vi "Digital Patterns Page.vi"(8 "error in (no error)":errorcluster, 11 "Node Ptr":T1 format="%.0x") -> (0 "error out":errorcluster)   [LabVIEW 2015, in "Engine Simulation Toolkit System Explorer.lvlib"]
uses:
  Engine Simulation Toolkit System Explorer.lvlib
  <vilib>/NI Veristand/Custom Device API/Custom Device Item Ref.ctl
  Digital Patterns Page Data.ctl
  Digital Pattern.ctl
  Digital Pattern Base.ctl
  Digital Pattern Remove Edge.ctl
  Digital Pattern Add Pulse.ctl
  File Formats.lvlibp/Parent/EST Pattern.ctl
  Shared/Properties.vi
  Shared/Constants and GUIDs.vi
  <vilib>/NI Veristand/Custom Device API/Custom Device API.lvlib
  Shared/Engine Simulation Toolkit Shared.lvlib
  <vilib>/NI/GXML/GXML.lvlib
  File Formats.lvlibp/Parent/FileFormat.lvclass
panel:
  in  "FPGA Resource":u16(ring) items=["Select an item..."]
  in  "pattern_remove":bool
  in  "pattern_add":bool caption="remove_add"
  in  "add_add":bool caption="remove_add"
  in  "Chart_Offset":dbl caption="Offset" format="%#_6f"
  in  "Chart_Tooth":u16 caption="Tooth"
  in  "Chart_Position":dbl caption="Position" format="%#_6f"
  in  "Edge":bool
  in  "remove_Tooth":u16 caption="Start\nTooth"
  in  "add_Offset":dbl caption="Offset"
  in  "add_Width":dbl caption="Width"
  in  "add_Tooth":u16 caption="Tooth"
  in  "base_Offset":dbl caption="Offset"
  in  "base_Toothwidth":dbl caption="Tooth width"
  in  "base_teeth":u16 caption="Teeth"
  in  "base_Length":dbl caption="Length"
  in  "add_remove":bool
  in  "remove_remove":bool
  in  "remove_add":bool
  in  "Pattern Name":string caption="Name"
  in  "Edges Removed":i32(listbox)
  in  "Pulses Added":i32(listbox)
  in  "Patterns":i32[](listbox)
  in  "Zoom":cluster{dbl, dbl}(slide)={360.0, -360.0} scale=-360.0..360.0
  out "Pattern Plot":cluster{dbl[], dbl[]}[](graph)
  in  "Header":cluster{"Section Name":string}={"Section Name"="Digital Patterns Settings"}
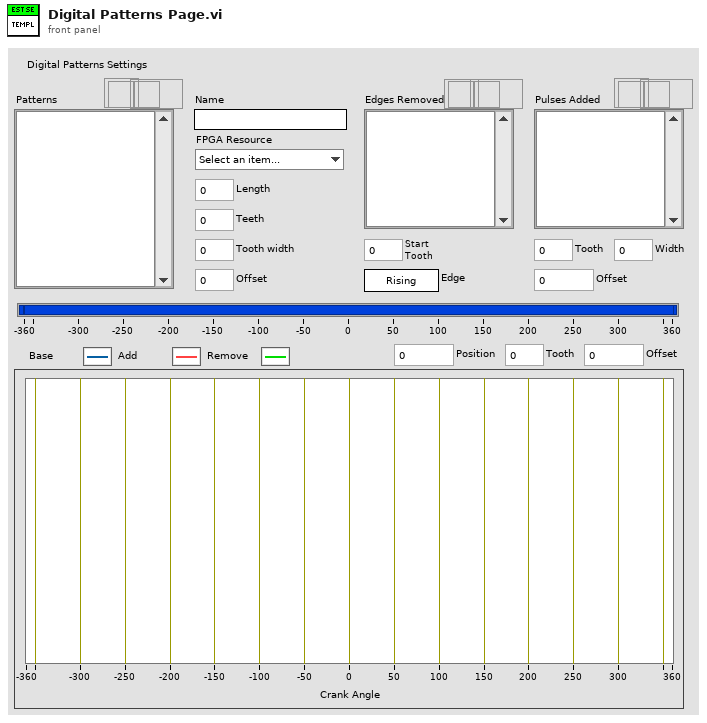
[diagram p1: front panel]
types:
  T1 = typedef "Custom Device API.lvlib/Custom Device Item Ref.ctl" = u64
  T2 = typedef "Engine Simulation Toolkit System Explorer.lvlib/Digital Patterns Page Data.ctl" = cluster{"SysExp Event":refnum<event-registration>, "Init done":bool, "Node Ptr":T1, "Ctrl Refs":cluster{"Header":refnum<vi>, "Pattern Plot":refnum<vi>, "Zoom":refnum<vi>, "Select Pattern":refnum<vi>, "Add List":refnum<vi>, "Remove List":refnum<vi>, "Pattern Name":refnum<vi>, "remove_add":refnum<vi>, "remove_remove":refnum<vi>, "add_remove":refnum<vi>, "base_Length":refnum<vi>, "base_teeth":refnum<vi>, "base_Toothwidth":refnum<vi>, "base_Offset":refnum<vi>, "add_Tooth":refnum<vi>, "add_Width":refnum<vi>, "add_Offset":refnum<vi>, "remove_Tooth":refnum<vi>, "remove_Edge":refnum<vi>, "Chart_Position":refnum<vi>, "Chart_Tooth":refnum<vi>, "Chart_Offset":refnum<vi>, "add_add":refnum<vi>, "pattern_remove":refnum<vi>, "pattern_add":refnum<vi>, "FPGA Resource":refnum<vi>}, "SE ref":refnum<vi>, "Patterns":T3[], "Sel patterns":i32[], "rotations":u16, "Need save":bool, "Rem List":i32, "Add List":i32, "FPGA Resources":string[]}
  T3 = typedef "Engine Simulation Toolkit System Explorer.lvlib/Digital Pattern.ctl" = cluster{"Name":string, "Base":T4, "Remove":T5[], "Add":T6[], "FPGA Resource":string}
  T4 = typedef "Engine Simulation Toolkit System Explorer.lvlib/Digital Pattern Base.ctl" = cluster{"Length":dbl, "Teeth":u16, "Width":dbl, "Offset":dbl}
  T5 = typedef "Engine Simulation Toolkit System Explorer.lvlib/Digital Pattern Remove Edge.ctl" = cluster{"Tooth":u16, "Edge":bool}
  T6 = typedef "Engine Simulation Toolkit System Explorer.lvlib/Digital Pattern Add Pulse.ctl" = cluster{"Tooth":u16, "Offset":dbl, "Width":dbl}
  T7 = typedef "Custom Device API.lvlib/Custom Device Commands.ctl" = enum16{"Default", "Item renamed", "Shutdown", "Dynamic button pressed"}
  T8 = typedef "LVPoint32TypeDef.ctl" = cluster{"Horizontal":i32, "Vertical":i32}
  T9 = typedef "File Formats.lvlibp/FileFormat.lvclass/EST Pattern.ctl" = cluster{"Base":cluster{"Length":dbl, "Teeth":u16, "Width":dbl, "Offset":dbl}, "Remove":cluster{"Tooth":u16, "Edge":bool}[], "Add":cluster{"Tooth":u16, "Offset":dbl, "Width":dbl}[]}
  T10 = cluster{"Length":dbl, "Teeth":u16, "Width":dbl, "Offset":dbl}
  T11 = cluster{"Tooth":u16, "Offset":dbl, "Width":dbl}[]
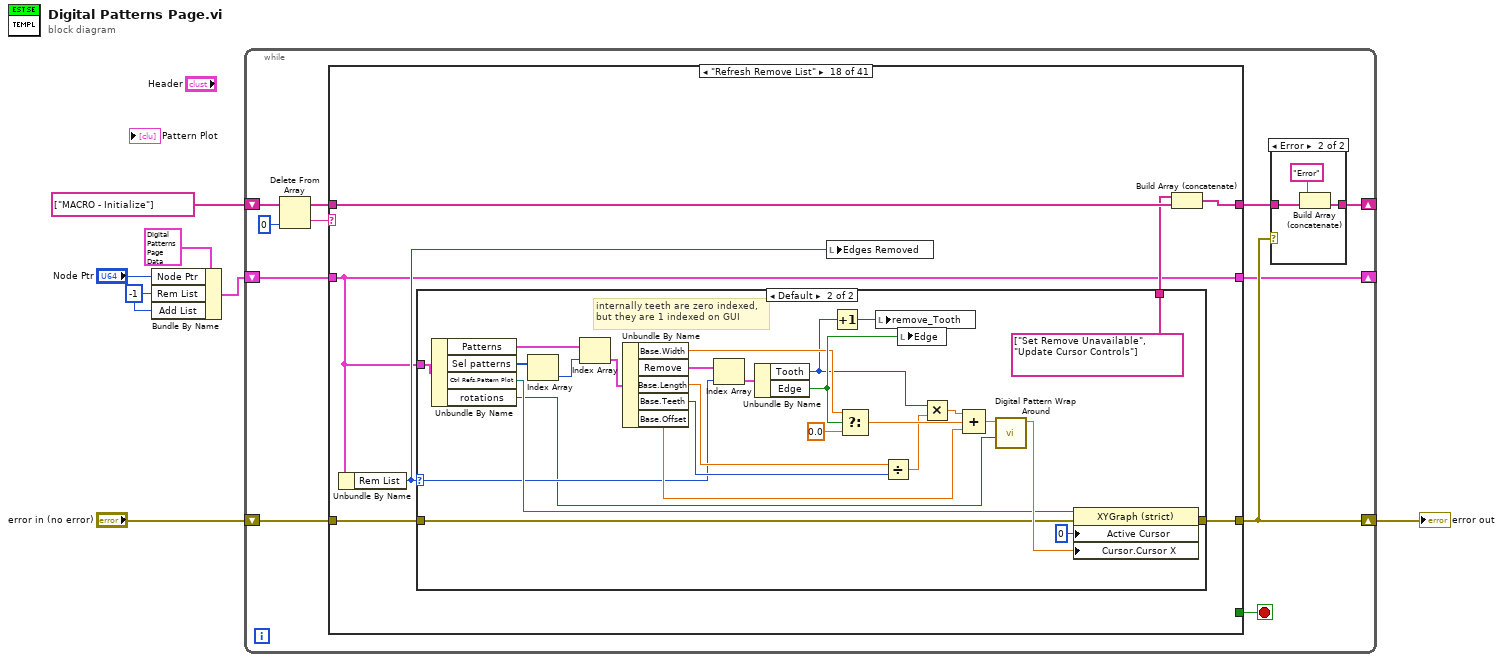
[diagram p0: block diagram]
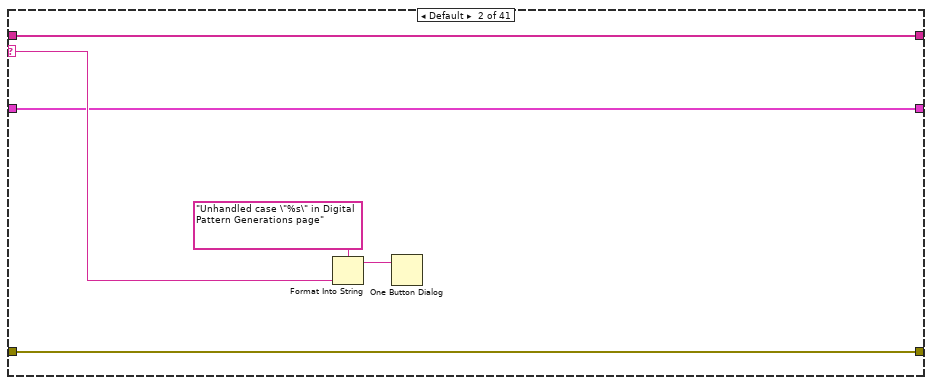
[diagram p4: hidden frame]
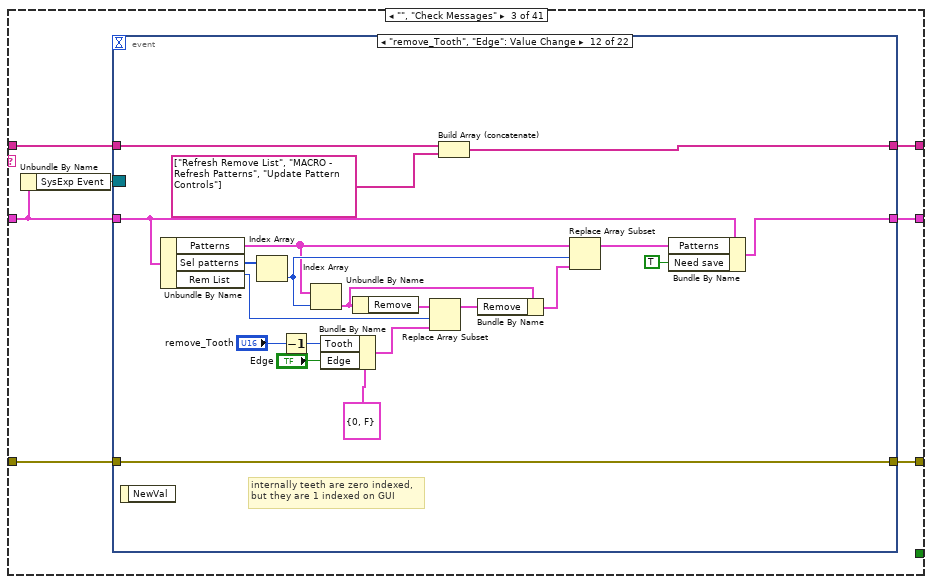
[diagram p5: hidden frame]
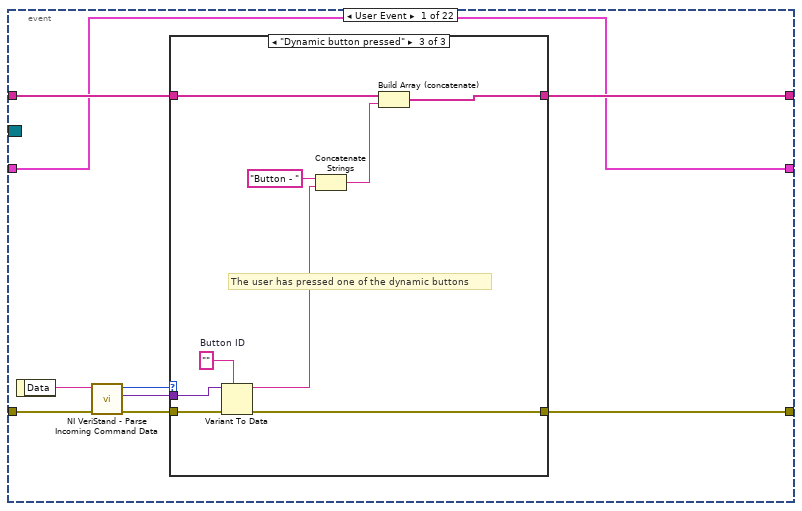
[diagram p6: hidden frame]
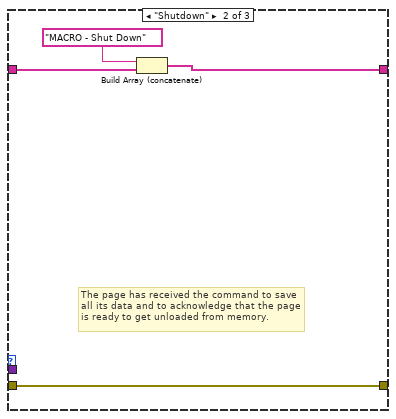
[diagram p8: hidden frame]
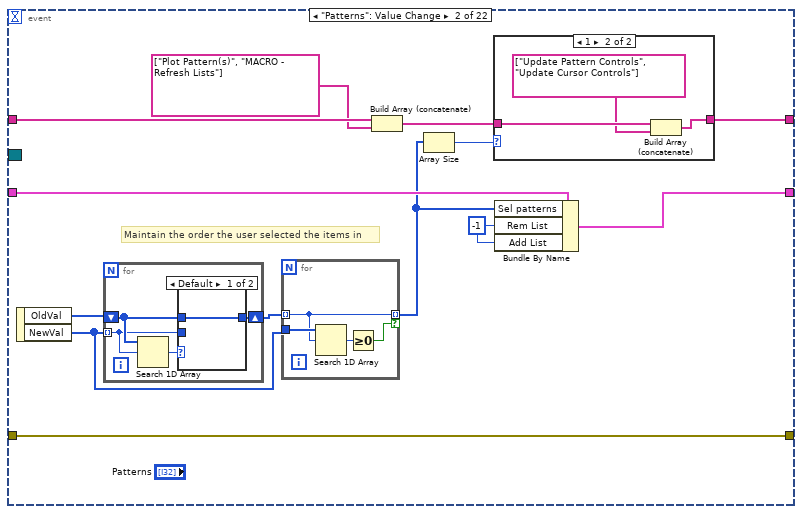
[diagram p9: hidden frame]
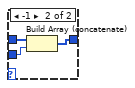
[diagram p11: hidden frame]
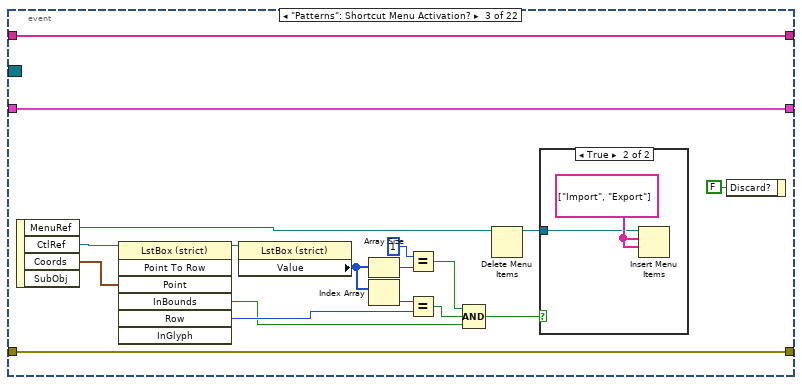
[diagram p12: hidden frame]
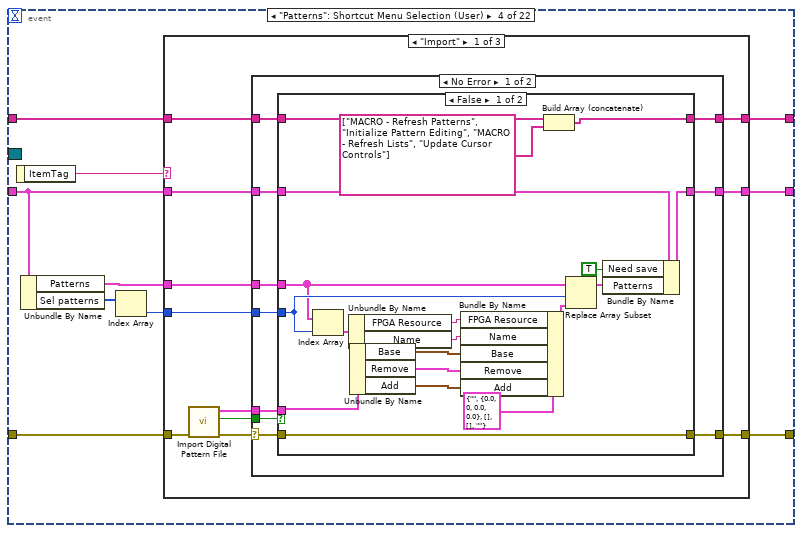
[diagram p14: hidden frame]
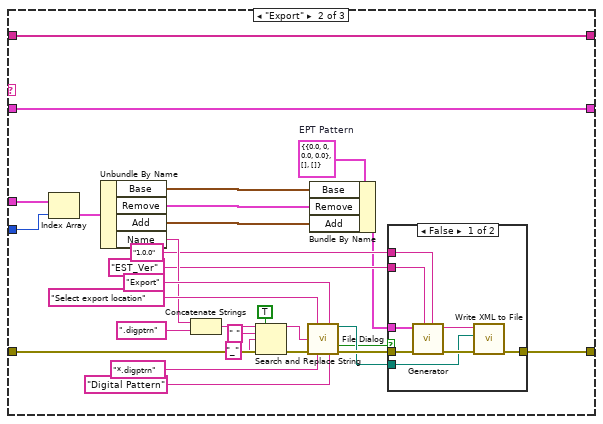
[diagram p17: hidden frame]
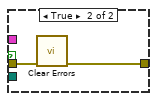
[diagram p18: hidden frame]
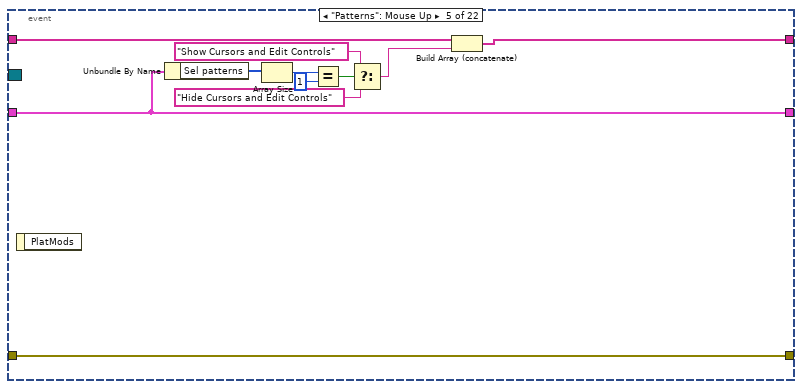
[diagram p20: hidden frame]
diagram:
  w1 = -1 ("Rem List")
  n1 = Bundle By Name(cluster=T2 {"SysExp Event"=refnum, "Init done"=FALSE, "Node Ptr"=0, "Ctrl Refs"={"Header"=refnum, "Pattern Plot"=refnum, "Zoom"=refnum, "Select Pattern"=refnum, "Add List"=refnum, "Remove List"=refnum, "Pattern Name"=refnum, "remove_add"=refnum, "remove_remove"=refnum, "add_remove"=refnum, "base_Length"=refnum, "base_teeth"=refnum, "base_Toothwidth"=refnum, "base_Offset"=refnum, "add_Tooth"=refnum, "add_Width"=refnum, "add_Offset"=refnum, "remove_Tooth"=refnum, "remove_Edge"=refnum, "Chart_Position"=refnum, "Chart_Tooth"=refnum, "Chart_Offset"=refnum, "add_add"=refnum, "pattern_remove"=refnum, "pattern_add"=refnum, "FPGA Resource"=refnum}, "SE ref"=refnum, "Patterns"=[], "Sel patterns"=[], "rotations"=0, "Need save"=FALSE, "Rem List"=0, "Add List"=0, "FPGA Resources"=[]} ("Page Data"), "Node Ptr"="Node Ptr", "Rem List"=w1, "Add List"=w1) -> (w3:T2)
  n2 = while {
    shift-right: [w13] -> _
    shift-left: string[] ["MACRO - Initialize"] -> [w18]
    shift-right: [w10] -> w5
    shift-left: "error in (no error)" -> [w12]
    shift-right: [w9] -> _
    shift-left: w3 -> [w14]
    stop <- w16 stop-if-true
    n3 = Delete From Array(array=w18, index=0) -> (deleted portion=w8:string, array with subset deleted=w17:string[])  [unwired: 1 in]
    n4 = case shown="\"Refresh Remove List\"" w8 {
      selector: w8 -> [_ w30 _ _ _ _ _ _ _ _ _ _ _ _ _ _ _ _ _ _ _ _ _ _ _ _ _ _ _ _ _ _ _ _ _ _ _ _ _ _ _]
      tunnel: [w23 w26 w38 w507 w521 w525 w528 w544 w553 w558 w562 w573 w591 w602 w614 w626 w630 w667 w724 w749 w764 w765 w774 w788 w789 w793 w796 w803 w808 w813 w816 w846 w852 w860 w867 w872 w879 w895 w907 w914 w919] -> w15
      tunnel: w17 -> [w23 w26 w37 w508 w521 w525 w528 w544 w553 w558 w562 w573 w591 w602 w614 w626 w637 w670 w724 w749 w764 w765 w774 w788 w789 w793 w797 w804 w809 w814 w816 w846 w852 w860 w867 w872 w879 w895 w907 w914 w920]
      tunnel: [_ _ _ _ _ _ _ _ _ _ _ _ _ _ _ _ _ _ _ _ _ _ _ _ TRUE _ _ _ _ _ _ _ _ _ _ _ _ _ _ _ _] -> w16
      tunnel: w12 -> [w25 w28 w35 w512 w520 w524 w527 w531 w552 w557 w561 w572 w590 w601 w613 w625 w633 w669 w723 w748 w763 w767 w773 w782 w791 w795 w800 w805 w810 w815 w818 w845 w850 w857 w864 w871 w878 w894 w906 w913 w916]
      tunnel: [w25 w28 w32 errorcluster {"status"=FALSE, "code"=0, "source"=""} ("error constant") w519 w524 w527 w531 w551 w555 w560 w567 w590 w601 w613 w625 w632 w668 w723 w748 w763 w767 w771 w783 w791 w795 w800 w805 w810 w815 w818 w845 w849 w856 w863 w871 w874 w883 w900 w913 w916] -> w10
      tunnel: w14 -> [w24 w27 w34 w510 w518 w523 w526 w534 w550 w554 w559 w571 w589 w600 w612 w624 w631 w664 w722 w747 w762 w766 w772 w787 w790 w794 w799 w802 w807 w812 w817 w848 w851 w855 w866 w870 w877 w893 w904 w912 w917]
      tunnel: [w24 w27 w36 w510 w518 w523 w526 w534 w550 w554 w559 w564 w589 w600 w612 w624 w631 w664 w722 w747 w762 w766 w772 w787 w790 w794 w799 w802 w807 w812 w817 w847 w851 w853 w862 w869 w875 w892 w901 w910 w917] -> w9
      frame "<------------------ System ------------------>" {
      }
      frame Default {
        n5 = Format Into String(format string="Unhandled case \"%s\" in Digital Pattern Generations page", w30) -> (resulting string=w31:string)  [unwired: 2 in, 1 out]
        n6 = One Button Dialog(message=w31) -> ()  [unwired: 1 in, 1 out]
      }
      frame "", "Check Messages" {
        n7 = Unbundle By Name(w34) -> ("SysExp Event"=w33:refnum<event-registration>)
        n8 = event shown="[11] \"remove_Tooth\", \"Edge\": Value Change" {
          selector: w33 -> [_ _ _ _ _ _ _ _ _ _ _ _ _ _ _ _ _ _ _ _ _ _]
          dyn-events: _ -> [_ _ _ _ _ _ _ _ _ _ _ _ _ _ _ _ _ _ _ _ _ _]
          timeout: _ -> [_ _ _ _ _ _ _ _ _ _ _ _ _ _ _ _ _ _ _ _ _ _]
          tunnel: [w40 w66 w109 w113 w213 w223 w229 w242 w250 w266 w274 w317 w339 w352 w360 w383 w398 w406 w410 w430 w458 w495] -> w38
          tunnel: w37 -> [w41 w75 w109 w112 w214 w226 w232 w242 w260 w261 w275 w325 w347 w353 w361 w384 w399 w407 w427 w447 w469 w506]
          tunnel: [w39 w70 w108 w117 w219 w224 w230 w241 w252 w267 w276 w319 w341 w350 w359 w382 w394 w402 w413 w433 w460 w497] -> w36
          tunnel: w34 -> [w39 w74 w108 w116 w219 w225 w231 w241 w253 w268 w291 w320 w342 w355 w379 w391 w396 w404 w425 w445 w467 w504]
          tunnel: w35 -> [w47 w69 w107 w115 w220 w222 w228 w240 w259 w262 w281 w324 w346 w354 w377 w389 w395 w403 w426 w446 w468 w505]
          tunnel: [w42 w69 w107 w114 w220 w221 w227 w239 w259 w263 w282 w324 w346 w354 w363 w386 w395 w403 w426 w446 w468 w505] -> w32
          event User Event {
            n9 = event-data() -> ("Data"=w46:string)  [unwired: 1 in]
            n10 = call <vilib>:"NI VeriStand - Parse Incoming Command Data.vi"("error in (no error)"=w47, "Incoming data"=w46) -> ("error out"=w44:errorcluster, "Outgoing data"=w43:variant, "Action"=w45:T7)  [unwired: 7 out]
            n11 = case shown="\"Dynamic button pressed\"" w45 {
              tunnel: [w49 w53 w61] -> w42
              tunnel: w44 -> [w49 w53 w60]
              tunnel: w43 -> [_ _ w59]
              tunnel: w41 -> [w48 w52 w58]
              tunnel: [w48 w50 w57] -> w40
              frame "Default", Default {
              }
              frame "Shutdown" {
                # "The page has received the command to save all its data and to acknowledge that the page is ready to get unloaded from memory."
                n12 = Build Array (concatenate)("MACRO - Shut Down", w52) -> (w50:string[])
              }
              frame "Dynamic button pressed" {
                w62 = ""  # Button ID
                # "The user has pressed one of the dynamic buttons"
                n13 = Variant To Data(error in=w60, type=w62, Variant=w59) -> (data=w55:string, error out=w61:errorcluster)
                n14 = Concatenate Strings("Button - " ("string"), w55) -> (w54:string)
                n15 = Build Array (concatenate)(w58, w54) -> (w57:string[])
              }
            }
          }
          event "Patterns": Value Change {
            w63 = -1 ("Rem List")
            # "Maintain the order the user selected the items in"
            n16 = event-data() -> ("OldVal"=w71:i32[], "NewVal"=w72:i32[])  [unwired: 1 in]
            n17 = for {
              tunnel: w72 -> [w84] mode=indexing
              shift-right: [w85] -> w73
              shift-left: w71 -> [w86]
              n18 = Search 1D Array(1D array=w86, element=w84) -> (index of element=w87:i32)  [unwired: 1 in]
              n19 = case shown="Default" w87 {
                tunnel: w86 -> [w88 w91]
                tunnel: [w88 w90] -> w85
                tunnel: w84 -> [_ w89]
                frame Default {
                }
                frame -1 {
                  n20 = Build Array (concatenate)(w91, w89) -> (w90:i32[])
                }
              }
            }
            n21 = for {
              tunnel: w72 -> [w81]
              tunnel: w73 -> [w80] mode=indexing
              tunnel: [w80] -> w65 mode=indexing if=w82
              n22 = Search 1D Array(1D array=w81, element=w80) -> (index of element=w83:i32)  [unwired: 1 in]
              n23 = Greater Or Equal To 0?(x=w83) -> (x >= 0?=w82:bool)
            }
            n24 = Build Array (concatenate)(w75, string[] ["Plot Pattern(s)", "MACRO - Refresh Lists"]) -> (w68:string[])
            n25 = Array Size(array=w65) -> (size(s)=w64:i32)
            n26 = case shown="1" w64 {
              tunnel: w68 -> [w76 w79]
              tunnel: [w76 w78] -> w66
              frame Default {
              }
              frame 1 {
                n27 = Build Array (concatenate)(w79, string[] ["Update Pattern Controls", "Update Cursor Controls"]) -> (w78:string[])
              }
            }
            n28 = Bundle By Name(cluster=w74, "Sel patterns"=w65, "Rem List"=w63, "Add List"=w63) -> (w70:T2)
          }
          event "Patterns": Shortcut Menu Activation? {
            n29 = event-data() -> ("MenuRef"=w93:refnum<k9>, "CtlRef"=w105:refnum<vi>, "Coords"=w106:T8)  [unwired: 1 in, 1 out]
            n30 = invoke class="LstBox (strict)" method="Point To Row"(reference=w105, "Point"=w106) -> (reference out=w104:refnum<vi>, "InBounds"=w97:bool, "Row"=w98:i32)  [unwired: 5 in, 4 out]
            n31 = property class="LstBox (strict)"(reference=w104) -> ("Value"=w102:i32[])  [unwired: 1 in, 2 out]
            n32 = Array Size(array=w102) -> (size(s)=w101:i32)
            n33 = Index Array(array=w102) -> (element=w99:i32)  [unwired: 1 in]
            n34 = Equal?(x=1 ("y"), y=w101) -> (x = y?=w95:bool)
            n35 = Equal?(x=w99, y=w98) -> (x = y?=w96:bool)
            n36 = Compound Arithmetic op=AND(w95, w96, w97) -> (w94:bool)
            n37 = Delete Menu Items(9:w93) -> (3:w92:refnum<k9>)  [unwired: 3 in, 1 out]
            n38 = case shown="True" w94 {
              tunnel: w92 -> [_ w110]
              frame False {
              }
              frame True {
                w111 = string[] ["Import", "Export"] ("item names")
                n39 = Insert Menu Items(7:w111, 8:w111, 9:w110) -> ()  [unwired: 3 in, 3 out]
              }
            }
            n40 = event-data("Discard?"=FALSE) -> ()  [unwired: 1 in, 1 out]
          }
          event "Patterns": Shortcut Menu Selection (User) {
            n41 = event-data() -> ("ItemTag"=w118:string)  [unwired: 1 in]
            n42 = Unbundle By Name(w116) -> ("Patterns"=w119:T3[], "Sel patterns"=w120:i32[])
            n43 = Index Array(array=w120) -> (element=w121:i32)  [unwired: 1 in]
            n44 = case shown="\"Import\"" w118 {
              tunnel: w121 -> [w130 w196 _]
              tunnel: w119 -> [w123 w195 _]
              tunnel: [w131 w194 w209] -> w117
              tunnel: w116 -> [w132 w194 w209]
              tunnel: w115 -> [w126 w175 w208]
              tunnel: [w129 w193 w208] -> w114
              tunnel: [w128 w185 w207] -> w113
              tunnel: w112 -> [w127 w185 w207]
              frame "Import" {
                n45 = call "Import Digital Pattern File.vi"("error in (no error)"=w126) -> ("error out"=w122:errorcluster, "Canceled?"=w125:bool, "EPT Pattern"=w124:T9)  [unwired: 8 in]
                n46 = case shown="No Error" w122 {
                  selector: w122 -> [w133 w167]
                  tunnel: w132 -> [w142 w166]
                  tunnel: [w141 w166] -> w131
                  tunnel: w130 -> [w140 _]
                  tunnel: [w139 w167] -> w129
                  tunnel: [w138 w165] -> w128
                  tunnel: w127 -> [w137 w165]
                  tunnel: w125 -> [w136 _]
                  tunnel: w124 -> [w135 _]
                  tunnel: w123 -> [w134 _]
                  frame No Error {
                    n47 = case shown="False" w136 {
                      tunnel: w142 -> [w161 w164]
                      tunnel: [w160 w164] -> w141
                      tunnel: w134 -> [w151 _]
                      tunnel: w140 -> [w152 _]
                      tunnel: w133 -> [w159 w162]
                      tunnel: [w159 w162] -> w139
                      tunnel: [w158 w163] -> w138
                      tunnel: w137 -> [w157 w163]
                      tunnel: w135 -> [w150 _]
                      frame False {
                        n48 = Index Array(array=w151, index=w152) -> (element=w155:T3)
                        n49 = Unbundle By Name(w155) -> ("FPGA Resource"=w154:string, "Name"=w153:string)
                        n50 = Unbundle By Name(w150) -> ("Base"=w145:T10, "Remove"=w144:cluster{"Tooth":u16, "Edge":bool}[], "Add"=w143:T11)
                        n51 = Bundle By Name(cluster=T3 {"Name"="", "Base"={"Length"=0.0, "Teeth"=0, "Width"=0.0, "Offset"=0.0}, "Remove"=[], "Add"=[], "FPGA Resource"=""} ("element"), "FPGA Resource"=w154, "Name"=w153, "Base"=w145, "Remove"=w144, "Add"=w143) -> (w147:T3)
                        n52 = Build Array (concatenate)(w157, string[] ["MACRO - Refresh Patterns", "Initialize Pattern Editing", "MACRO - Refresh Lists", "Update Cursor Controls"]) -> (w158:string[])
                        n53 = Replace Array Subset(array=w151, new element=w147, index=w152) -> (w149:T3[])
                        n54 = Bundle By Name(cluster=w161, "Need save"=TRUE, "Patterns"=w149) -> (w160:T2)
                      }
                      frame True {
                      }
                    }
                  }
                  frame Error {
                  }
                }
              }
              frame "Export" {
                w168 = T9 {"Base"={"Length"=0.0, "Teeth"=0, "Width"=0.0, "Offset"=0.0}, "Remove"=[], "Add"=[]}  # EPT Pattern
                n55 = Index Array(array=w195, index=w196) -> (element=w187:T3)
                n56 = Unbundle By Name(w187) -> ("Base"=w179:T4, "Remove"=w178:T5[], "Add"=w177:T6[], "Name"=w186:string)
                n57 = Concatenate Strings(w186, ".digptrn" ("button label")) -> (w172:string)
                n58 = Search and Replace String(replace all?=TRUE ("replace all? (F)"), input string=w172, search string=" ", replace string="_" ("replace string (\"\")"), error in=w175) -> (result string=w173:string, error out=w174:errorcluster)  [unwired: 3 in, 2 out]
                n59 = call "File Dialog"("prompt"="Select export location", "button label"="Export", "default name"=w173, "error in"=w174, "pattern (all files)"="*.digptrn" ("button label"), "pattern label"="Digital Pattern" ("button label")) -> ("selected path"=w190:path, "cancelled"=w189:bool, "error out"=w192:errorcluster)  [unwired: 6 in, 1 out]
                n60 = Bundle By Name(cluster=w168, "Base"=w179, "Remove"=w178, "Add"=w177) -> (w176:T9)
                n61 = case shown="False" w189 {
                  tunnel: w176 -> [w204 _]
                  tunnel: [w201 w205] -> w193
                  tunnel: w192 -> [w200 w206]
                  tunnel: w190 -> [w199 _]
                  tunnel: "EST_Ver" ("prompt") -> [w198 _]
                  tunnel: "1.0.0" ("button label") -> [w197 _]
                  frame False {
                    n62 = call <vilib>:"Generator.vi"("Version String"=w197, "Version Tag Name"=w198, "error in"=w200, "Variant"=w204) -> ("error out"=w202:errorcluster, "XML String Out"=w203:string)  [unwired: 6 in]
                    n63 = call <vilib>:"Write XML to File.vi"("error in"=w202, "XML File Path"=w199, "XML Input"=w203) -> ("error out"=w201:errorcluster)  [unwired: 8 in]
                  }
                  frame True {
                    n64 = call <vilib>:"Clear Errors.vi"("error in (no error)"=w206) -> ("error out"=w205:errorcluster)  [unwired: 5 in, 1 out]
                  }
                }
              }
              frame Default {
              }
            }
          }
          event "Patterns": Mouse Up {
            n65 = event-data() -> ()  [unwired: 1 in, 1 out]
            n66 = Unbundle By Name(w219) -> ("Sel patterns"=w218:i32[])
            n67 = Array Size(array=w218) -> (size(s)=w217:i32)
            n68 = Equal?(x=w217, y=1) -> (x = y?=w215:bool)
            n69 = Select(t="Show Cursors and Edit Controls", s=w215, f="Hide Cursors and Edit Controls") -> (s? t:f=w210:string)
            n70 = Build Array (concatenate)(w214, w210) -> (w213:string[])
          }
          event "pattern_remove": Value Change {
            n71 = event-data() -> ()  [unwired: 1 in, 1 out]
            n72 = call "Remove Digital Pattern.vi"("error in (no error)"=w222, "Page Data in"=w225, "State queue in"=w226) -> ("error out"=w221:errorcluster, "Page Data out"=w224:T2, "State queue out"=w223:string[])  [unwired: 6 in]
          }
          event "pattern_add": Value Change {
            n73 = event-data() -> ()  [unwired: 1 in, 1 out]
            n74 = call "Add Digital Pattern.vi"("error in (no error)"=w228, "Page Data in"=w231, "State queue in"=w232) -> ("error out"=w227:errorcluster, "Page Data out"=w230:T2, "State queue out"=w229:string[])  [unwired: 6 in]
          }
          event "Zoom": Value Change {
            n75 = event-data() -> ("NewVal"=w235:cluster{dbl, dbl})  [unwired: 1 in]
            n76 = Unbundle By Name(w241) -> ("Ctrl Refs.Pattern Plot"=w238:refnum<vi>)
            n77 = Unbundle(w235) -> (w237:dbl, w236:dbl)
            n78 = Max & Min(x=w237, y=w236) -> (max(x,y)=w234:dbl, min(x,y)=w233:dbl)
            n79 = property on="Property Node" class="XYGraph (strict)"(reference=w238, error in=w240, "XScale.Maximum"=w234, "XScale.Minimum"=w233) -> (error out=w239:errorcluster)  [unwired: 1 out]
          }
          event "base_Length", "base_teeth", "base_Toothwidth", "base_Offset": Value Change {
            n80 = event-data() -> ()  [unwired: 1 in, 6 out]
            n81 = Unbundle By Name(w253) -> ("Patterns"=w255:T3[], "Sel patterns"=w254:i32[])
            n82 = Index Array(array=w254) -> (element=w256:i32)  [unwired: 1 in]
            n83 = Build Array (concatenate)(w260, "Plot Pattern(s)", "Update Cursor Controls") -> (w250:string[])
            n84 = Index Array(array=w255, index=w256) -> (element=w257:T3)
            n85 = Bundle By Name(cluster=w257, "Base.Length"="base_Length", "Base.Teeth"="base_teeth", "Base.Width"="base_Toothwidth", "Base.Offset"="base_Offset") -> (w258:T3)
            n86 = Replace Array Subset(array=w255, new element=w258, index=w256) -> (w251:T3[])
            n87 = Bundle By Name(cluster=w253, "Patterns"=w251, "Need save"=TRUE) -> (w252:T2)
          }
          event "Pattern Name": Value Change {
            n88 = event-data() -> ("NewVal"=w264:string, "OldVal"=w265:string)  [unwired: 1 in]
            n89 = call "Rename Digital Pattern.vi"("OldVal"=w265, "error in (no error)"=w262, "NewVal"=w264, "Page Data in"=w268, "State Queue in"=w261) -> ("error out"=w263:errorcluster, "Page Data out"=w267:T2, "State Queue out"=w266:string[])  [unwired: 4 in]
          }
          event "FPGA Resource": Value Change {
            n90 = event-data() -> ("OldVal"=w286:u16, "NewVal"=w269:u16)  [unwired: 1 in]
            n91 = Unbundle By Name(w291) -> ("Patterns"=w292:T3[], "Sel patterns"=w288:i32[], "FPGA Resources"=w287:string[])
            n92 = Decrement(x=w286) -> (x-1=w285:u16)
            n93 = Decrement(x=w269) -> (x-1=w270:u16)
            n94 = Index Array(array=w287, index #1=w285, index #2=w270) -> (element #1=w278:string, element #2=w272:string)
            n95 = Index Array(array=w288) -> (element=w293:i32)  [unwired: 1 in]
            n96 = Index Array(array=w292, index=w293) -> (element=w284:T3)
            n97 = Bundle By Name(cluster=w284, "FPGA Resource"=w272) -> (w279:T3)
            n98 = Unbundle By Name(w284) -> ("Name"=w283:string)
            n99 = Equal?(x=w283, y=w278) -> (x = y?=w280:bool)
            n100 = Replace Array Subset(array=w292, new element=w279, index=w293) -> (w290:T3[])
            n101 = Not Equal To 0?(x=w269) -> (x != 0?=w271:bool)
            n102 = And(x=w280, y=w271) -> (x .and. y?=w273:bool)
            n103 = Bundle By Name(cluster=w291, "Patterns"=w290, "Need save"=TRUE) -> (w277:T2)
            n104 = case shown="True" w273 {
              tunnel: [w296 w303] -> w282
              tunnel: w281 -> [w296 w304]
              tunnel: w278 -> [_ w302]
              tunnel: w272 -> [_ w301]
              tunnel: w277 -> [w294 w300]
              tunnel: [w294 w299] -> w276
              tunnel: w275 -> [w295 w298]
              tunnel: [w295 w297] -> w274
              frame False {
              }
              frame True {
                n105 = call "Rename Digital Pattern.vi"("OldVal"=w302, "error in (no error)"=w304, "NewVal"=w301, "Page Data in"=w300, "State Queue in"=w298) -> ("error out"=w303:errorcluster, "Page Data out"=w299:T2, "State Queue out"=w297:string[])  [unwired: 4 in]
              }
            }
          }
          event "remove_Tooth", "Edge": Value Change {
            # "internally teeth are zero indexed, but they are 1 indexed on GUI"
            n106 = event-data() -> ()  [unwired: 1 in, 1 out]
            n107 = Unbundle By Name(w320) -> ("Patterns"=w322:T3[], "Sel patterns"=w321:i32[], "Rem List"=w314:i32)
            n108 = Index Array(array=w321) -> (element=w323:i32)  [unwired: 1 in]
            n109 = Decrement(x="remove_Tooth") -> (x-1=w305:u16)
            n110 = Index Array(array=w322, index=w323) -> (element=w308:T3)
            n111 = Bundle By Name(cluster=T5 {"Tooth"=0, "Edge"=FALSE} ("Cluster"), "Tooth"=w305, "Edge"="Edge") -> (w310:T5)
            n112 = Unbundle By Name(w308) -> ("Remove"=w315:T5[])
            n113 = Replace Array Subset(array=w315, new element=w310, index=w314) -> (w309:T5[])
            n114 = Build Array (concatenate)(w325, string[] ["Refresh Remove List", "MACRO - Refresh Patterns", "Update Pattern Controls"]) -> (w317:string[])
            n115 = Bundle By Name(cluster=w308, "Remove"=w309) -> (w307:T3)
            n116 = Replace Array Subset(array=w322, new element=w307, index=w323) -> (w318:T3[])
            n117 = Bundle By Name(cluster=w320, "Patterns"=w318, "Need save"=TRUE) -> (w319:T2)
          }
          event "add_Tooth", "add_Width", "add_Offset": Value Change {
            # "internally teeth are zero indexed, but they are 1 indexed on GUI"
            n118 = event-data() -> ()  [unwired: 1 in, 3 out]
            n119 = Unbundle By Name(w342) -> ("Patterns"=w344:T3[], "Sel patterns"=w343:i32[], "Add List"=w336:i32)
            n120 = Index Array(array=w343) -> (element=w345:i32)  [unwired: 1 in]
            n121 = Decrement(x="add_Tooth") -> (x-1=w326:u16)
            n122 = Index Array(array=w344, index=w345) -> (element=w332:T3)
            n123 = Bundle By Name(cluster=T6 {"Tooth"=0, "Offset"=0.0, "Width"=0.0} ("Cluster"), "Tooth"=w326, "Offset"="add_Offset", "Width"="add_Width") -> (w334:T6)
            n124 = Unbundle By Name(w332) -> ("Add"=w337:T6[])
            n125 = Replace Array Subset(array=w337, new element=w334, index=w336) -> (w333:T6[])
            n126 = Build Array (concatenate)(w347, string[] ["Refresh Add List", "MACRO - Refresh Patterns", "Update Pattern Controls"]) -> (w339:string[])
            n127 = Bundle By Name(cluster=w332, "Add"=w333) -> (w331:T3)
            n128 = Replace Array Subset(array=w344, new element=w331, index=w345) -> (w340:T3[])
            n129 = Bundle By Name(cluster=w342, "Patterns"=w340, "Need save"=TRUE) -> (w341:T2)
          }
          event "Pattern Plot": Cursor Move {
            w349 = -1 ("Add List")
            n130 = event-data() -> ()  [unwired: 1 in, 1 out]
            n131 = Build Array (concatenate)(w353, "MACRO - Refresh Lists", "Update Cursor Controls") -> (w352:string[])
            n132 = Bundle By Name(cluster=w355, "Rem List"=w349, "Add List"=w349) -> (w350:T2)
          }
          event "Chart_Tooth", "Chart_Offset": Value Change {
            w358 = -1 ("Add List")
            # "internally teeth are zero indexed, but they are 1 indexed on GUI"
            n133 = event-data() -> ()  [unwired: 1 in, 1 out]
            n134 = Unbundle By Name(w379) -> ("Patterns"=w374:T3[], "Sel patterns"=w373:i32[], "Ctrl Refs.Pattern Plot"=w376:refnum<vi>)
            n135 = Index Array(array=w373) -> (element=w375:i32)  [unwired: 1 in]
            n136 = Index Array(array=w374, index=w375) -> (element=w372:T3)
            n137 = Unbundle By Name(w372) -> ("Base.Length"=w368:dbl, "Base.Teeth"=w369:u16, "Base.Offset"=w367:dbl)
            n138 = Decrement(x="Chart_Tooth") -> (x-1=w356:u16)
            n139 = Divide(x=w368, y=w369) -> (x/y=w370:dbl)
            n140 = Multiply(x=w356, y=w370) -> (x*y=w371:dbl)
            n141 = Compound Arithmetic op=ADD(w371, "Chart_Offset", w367) -> (w364:dbl)
            n142 = Build Array (concatenate)(w361, "MACRO - Refresh Lists", "Update Cursor Controls") -> (w360:string[])
            n143 = property on="Property Node" class="XYGraph (strict)"(reference=w376, error in=w377, "Active Cursor"=u32 0, "Cursor.Cursor X"=w364) -> (error out=w363:errorcluster)  [unwired: 1 out]
            n144 = Bundle By Name(cluster=w379, "Rem List"=w358, "Add List"=w358) -> (w359:T2)
          }
          event "Chart_Position": Value Change {
            w381 = -1 ("Add List")
            n145 = event-data() -> ("NewVal"=w387:dbl)  [unwired: 1 in]
            n146 = Unbundle By Name(w391) -> ("Ctrl Refs.Pattern Plot"=w388:refnum<vi>)
            n147 = property on="Property Node" class="XYGraph (strict)"(reference=w388, error in=w389, "Active Cursor"=u32 0, "Cursor.Cursor X"=w387) -> (error out=w386:errorcluster)  [unwired: 1 out]
            n148 = Build Array (concatenate)(w384, "MACRO - Refresh Lists", "Update Cursor Controls") -> (w383:string[])
            n149 = Bundle By Name(cluster=w391, "Rem List"=w381, "Add List"=w381) -> (w382:T2)
          }
          event "Edges Removed": Value Change {
            n150 = event-data() -> ("NewVal"=w393:i32)  [unwired: 1 in]
            n151 = Build Array (concatenate)(w399, "MACRO - Refresh Lists") -> (w398:string[])
            n152 = Bundle By Name(cluster=w396, "Rem List"=w393, "Add List"=-1) -> (w394:T2)
          }
          event "Pulses Added": Value Change {
            n153 = event-data() -> ("NewVal"=w400:i32)  [unwired: 1 in]
            n154 = Bundle By Name(cluster=w404, "Rem List"=-1 ("Add List"), "Add List"=w400) -> (w402:T2)
            n155 = Build Array (concatenate)(w407, "MACRO - Refresh Lists") -> (w406:string[])
          }
          event "remove_remove": Value Change {
            n156 = event-data() -> ()  [unwired: 1 in, 2 out]
            n157 = Unbundle By Name(w425) -> ("Patterns"=w417:T3[], "Sel patterns"=w424:i32[], "Rem List"=w414:i32)
            n158 = Index Array(array=w424) -> (element=w416:i32)  [unwired: 1 in]
            n159 = Index Array(array=w417, index=w416) -> (element=w415:T3)
            n160 = Unbundle By Name(w415) -> ("Remove"=w419:T5[])
            n161 = Delete From Array(array=w419, index=w414) -> (array with subset deleted=w423:T5[])  [unwired: 1 in, 1 out]
            n162 = Build Array (concatenate)(w427, string[] ["Refresh Remove List", "Update Pattern Controls", "MACRO - Refresh Patterns"]) -> (w410:string[])
            n163 = Array Size(array=w423) -> (size(s)=w420:i32)
            n164 = Bundle By Name(cluster=w415, "Remove"=w423) -> (w418:T3)
            n165 = Decrement(x=w420) -> (x-1=w421:i32)
            n166 = In Range and Coerce(upper limit=w421, x=w414, lower limit=-1) -> (coerced(x)=w411:i32)  [unwired: 1 out]
            n167 = Replace Array Subset(array=w417, new element=w418, index=w416) -> (w412:T3[])
            n168 = Bundle By Name(cluster=w425, "Patterns"=w412, "Rem List"=w411, "Need save"=TRUE) -> (w413:T2)
          }
          event "add_remove": Value Change {
            n169 = event-data() -> ()  [unwired: 1 in, 2 out]
            n170 = Unbundle By Name(w445) -> ("Patterns"=w437:T3[], "Sel patterns"=w444:i32[], "Add List"=w434:i32)
            n171 = Index Array(array=w444) -> (element=w436:i32)  [unwired: 1 in]
            n172 = Index Array(array=w437, index=w436) -> (element=w435:T3)
            n173 = Unbundle By Name(w435) -> ("Add"=w439:T6[])
            n174 = Delete From Array(array=w439, index=w434) -> (array with subset deleted=w443:T6[])  [unwired: 1 in, 1 out]
            n175 = Build Array (concatenate)(w447, string[] ["Refresh Add List", "Update Pattern Controls", "MACRO - Refresh Patterns"]) -> (w430:string[])
            n176 = Array Size(array=w443) -> (size(s)=w440:i32)
            n177 = Bundle By Name(cluster=w435, "Add"=w443) -> (w438:T3)
            n178 = Decrement(x=w440) -> (x-1=w441:i32)
            n179 = In Range and Coerce(upper limit=w441, x=w434, lower limit=-1) -> (coerced(x)=w431:i32)  [unwired: 1 out]
            n180 = Replace Array Subset(array=w437, new element=w438, index=w436) -> (w432:T3[])
            n181 = Bundle By Name(cluster=w445, "Patterns"=w432, "Add List"=w431, "Need save"=TRUE) -> (w433:T2)
          }
          event "remove_add": Value Change {
            # "internally teeth are zero indexed, but they are 1 indexed on GUI"
            n182 = event-data() -> ()  [unwired: 1 in, 2 out]
            n183 = Unbundle By Name(w467) -> ("Patterns"=w463:T3[], "Sel patterns"=w466:i32[], "Rem List"=w449:i32)
            n184 = Index Array(array=w466) -> (element=w462:i32)  [unwired: 1 in]
            n185 = Index Array(array=w463, index=w462) -> (element=w461:T3)
            n186 = case shown="0, Default" w449 {
              selector: w449 -> [w475 _]
              tunnel: w461 -> [w476 w483]
              tunnel: [w472 w482] -> w455
              tunnel: [w474 w481] -> w454
              tunnel: [w470 w477] -> w448
              frame 0, Default {
                n187 = Unbundle By Name(w476) -> ("Remove"=w474:T5[])
                n188 = Index Array(array=w474, index=w475) -> (element=w473:T5)
                n189 = Unbundle By Name(w473) -> ("Edge"=w472:bool, "Tooth"=w471:u16)
                n190 = Increment(x=w471) -> (x+1=w470:u16)
              }
              frame -1 {
                n191 = Unbundle By Name(w483) -> ("Remove"=w481:T5[], "Base.Width"=w479:dbl)
                n192 = local read "Chart_Offset"() -> (w480:dbl)
                n193 = local read "Chart_Tooth"() -> (w478:u16)
                n194 = Less?(x=w479, y=w480) -> (x < y?=w482:bool)
                n195 = Decrement(x=w478) -> (x-1=w477:u16)
              }
            }
            n196 = Bundle By Name(cluster=T5 {"Tooth"=0, "Edge"=FALSE} ("Cluster"), "Edge"=w455, "Tooth"=w448) -> (w456:T5)
            n197 = Build Array (concatenate)(w469, string[] ["Refresh Remove List", "Update Pattern Controls", "MACRO - Refresh Patterns"]) -> (w458:string[])
            n198 = Build Array (concatenate)(w454, w456) -> (w453:T5[])
            n199 = Array Size(array=w453) -> (size(s)=w465:i32)
            n200 = Bundle By Name(cluster=w461, "Remove"=w453) -> (w464:T3)
            n201 = Decrement(x=w465) -> (x-1=w452:i32)
            n202 = Replace Array Subset(array=w463, new element=w464, index=w462) -> (w459:T3[])
            n203 = Bundle By Name(cluster=w467, "Patterns"=w459, "Rem List"=w452, "Need save"=TRUE) -> (w460:T2)
          }
          event "add_add": Value Change {
            # "internally teeth are zero indexed, but they are 1 indexed on GUI"
            n204 = event-data() -> ()  [unwired: 1 in, 2 out]
            n205 = Unbundle By Name(w504) -> ("Patterns"=w500:T3[], "Sel patterns"=w503:i32[])
            n206 = Index Array(array=w503) -> (element=w499:i32)  [unwired: 1 in]
            n207 = local read "Chart_Offset"() -> (w486:dbl)
            n208 = local read "Chart_Tooth"() -> (w491:u16)
            n209 = Index Array(array=w500, index=w499) -> (element=w498:T3)
            n210 = Unbundle By Name(w498) -> ("Add"=w492:T6[], "Base.Width"=w487:dbl)
            n211 = Decrement(x=w491) -> (x-1=w484:u16)
            n212 = Bundle By Name(cluster=T6 {"Tooth"=0, "Offset"=0.0, "Width"=0.0} ("Cluster"), "Width"=w487, "Offset"=w486, "Tooth"=w484) -> (w493:T6)
            n213 = Build Array (concatenate)(w492, w493) -> (w490:T6[])
            n214 = Build Array (concatenate)(w506, string[] ["Refresh Add List", "Update Pattern Controls", "MACRO - Refresh Patterns"]) -> (w495:string[])
            n215 = Array Size(array=w490) -> (size(s)=w502:i32)
            n216 = Bundle By Name(cluster=w498, "Add"=w490) -> (w501:T3)
            n217 = Decrement(x=w502) -> (x-1=w489:i32)
            n218 = Replace Array Subset(array=w500, new element=w501, index=w499) -> (w496:T3[])
            n219 = Bundle By Name(cluster=w504, "Patterns"=w496, "Add List"=w489, "Need save"=TRUE) -> (w497:T2)
          }
        }
      }
      frame "Error" {
        n220 = call <vilib>:"Simple Error Handler.vi"("error in (no error)"=w512) -> ()  [unwired: 4 in, 5 out]
        n221 = Unbundle By Name(w510) -> ("Init done"=w509:bool)
        n222 = case shown="False" w509 {
          tunnel: w508 -> [w515 w516]
          tunnel: [w514 w516] -> w507
          frame False {
            n223 = Build Array (concatenate)(string[] ["Release SE Cursor", "MACRO - Shut Down"], w515) -> (w514:string[])
          }
          frame True {
          }
        }
      }
      frame "Set Busy Cursor" {
        n224 = Unbundle By Name(w518) -> ("SE ref"=w517:refnum<vi>)
        n225 = call <vilib>:"Set Busy.vi"("error in (no error)"=w520, "VI reference (current VI)"=w517) -> ("error out"=w519:errorcluster)  [unwired: 8 in, 1 out]
      }
      frame "Clear Busy Cursor" {
        n226 = Unbundle By Name(w523) -> ("SE ref"=w522:refnum<vi>)
        n227 = call <vilib>:"Unset Busy.vi"("VI reference (current VI)"=w522) -> ()  [unwired: 10 in, 1 out]
      }
      frame "<------------- Front Panel Updates------------->" {
      }
      frame "Disable Add and Remove" {
        n228 = Unbundle By Name(w534) -> ("Ctrl Refs.Add List"=w532:refnum<vi>, "Ctrl Refs.Remove List"=w533:refnum<vi>, "Ctrl Refs.remove_add"=w543:refnum<vi>, "Ctrl Refs.remove_remove"=w542:refnum<vi>, "Ctrl Refs.add_remove"=w541:refnum<vi>, "Ctrl Refs.add_Tooth"=w540:refnum<vi>, "Ctrl Refs.add_Width"=w539:refnum<vi>, "Ctrl Refs.add_Offset"=w538:refnum<vi>, "Ctrl Refs.remove_Tooth"=w537:refnum<vi>, "Ctrl Refs.remove_Edge"=w536:refnum<vi>, "Ctrl Refs.add_add"=w529:refnum<vi>)
        n229 = Build Array(w532, w533, w543, w542, w541, w540, w539, w538, w537, w536, w529) -> (w530:refnum<vi>[])
        n230 = call "Enable_Disable Controls.vi"("Enable?"=FALSE ("Enabled?"), "Controls"=w530) -> ()  [unwired: 10 in]
      }
      frame "Plot Pattern(s)" {
        n231 = Unbundle By Name(w550) -> ("Ctrl Refs.Zoom"=w549:refnum<vi>, "Ctrl Refs.Pattern Plot"=w548:refnum<vi>, "Patterns"=w547:T3[], "rotations"=w546:u16, "Sel patterns"=w545:i32[])
        n232 = call "Expand Digital Pattern.vi"("Zoom"=w549, "Pattern Plot"=w548, "error in (no error)"=w552, "Select Patterns"=w545, "Rotations"=w546, "Patterns"=w547) -> ("error out"=w551:errorcluster)  [unwired: 5 in]
      }
      frame "Update Pattern Controls" {
        n233 = call "Update Digital Pattern Pattern Controls.vi"("error in (no error)"=w557, "Page Data in"=w554) -> ("error out"=w556:errorcluster)  [unwired: 9 in]
        n234 = call "Update Digital Pattern FPGA Resources.vi"("error in (no error)"=w556, "Page Data in"=w554) -> ("error out"=w555:errorcluster)  [unwired: 9 in]
      }
      frame "Update Cursor Controls" {
        n235 = call "Update Digital Pattern Cursor Controls.vi"("error in (no error)"=w561, "Page Data in"=w559) -> ("error out"=w560:errorcluster)  [unwired: 9 in]
      }
      frame "Populate Patterns List" {
        n236 = Unbundle By Name(w571) -> ("Patterns"=w569:T3[], "Sel patterns"=w568:i32[], "Ctrl Refs.Select Pattern"=w566:refnum<vi>)
        n237 = for {
          tunnel: w569 -> [w580] mode=indexing
          tunnel: [w579] -> w565 mode=indexing
          n238 = Unbundle By Name(w580) -> ("Name"=w579:string)
        }
        n239 = Array Size(array=w565) -> (size(s)=w570:i32)
        n240 = for {
          tunnel: w570 -> [w578]
          tunnel: [w576] -> w563 mode=indexing if=w574
          tunnel: w568 -> [w575] mode=indexing
          n241 = In Range and Coerce(upper limit=w578, x=w575, lower limit=0) -> (coerced(x)=w576:i32, In Range?=w574:bool)
        }
        n242 = property class="LstBox (strict)"(reference=w566, error in=w572, "Item Names"=w565, "Value"=w563) -> (error out=w567:errorcluster)  [unwired: 1 out]
        n243 = Bundle By Name(cluster=w571, "Sel patterns"=w563) -> (w564:T2)
      }
      frame "Set Remove Available" {
        n244 = Unbundle By Name(w589) -> ("Ctrl Refs.remove_add"=w584:refnum<vi>, "Ctrl Refs.remove_remove"=w588:refnum<vi>, "Ctrl Refs.remove_Tooth"=w586:refnum<vi>, "Ctrl Refs.remove_Edge"=w585:refnum<vi>)
        n245 = Build Array(w584) -> (w583:refnum<vi>[])
        n246 = Build Array(w588, w586, w585) -> (w587:refnum<vi>[])
        n247 = call "Enable_Disable Controls.vi"("Enable?"=TRUE, "Controls"=w583) -> ()  [unwired: 10 in]
        n248 = call "Enable_Disable Controls.vi"("Enable?"=FALSE, "Controls"=w587) -> ()  [unwired: 10 in]
      }
      frame "Set Remove Unavailable" {
        n249 = Unbundle By Name(w600) -> ("Ctrl Refs.remove_add"=w595:refnum<vi>, "Ctrl Refs.remove_remove"=w599:refnum<vi>, "Ctrl Refs.remove_Tooth"=w597:refnum<vi>, "Ctrl Refs.remove_Edge"=w596:refnum<vi>)
        n250 = Build Array(w595) -> (w594:refnum<vi>[])
        n251 = Build Array(w599, w597, w596) -> (w598:refnum<vi>[])
        n252 = call "Enable_Disable Controls.vi"("Enable?"=TRUE, "Controls"=w594) -> ()  [unwired: 10 in]
        n253 = call "Enable_Disable Controls.vi"("Enable?"=TRUE, "Controls"=w598) -> ()  [unwired: 10 in]
      }
      frame "Set Add Available" {
        n254 = Unbundle By Name(w612) -> ("Ctrl Refs.add_add"=w607:refnum<vi>, "Ctrl Refs.add_remove"=w611:refnum<vi>, "Ctrl Refs.add_Tooth"=w609:refnum<vi>, "Ctrl Refs.add_Width"=w608:refnum<vi>, "Ctrl Refs.add_Offset"=w604:refnum<vi>)
        n255 = Build Array(w607) -> (w606:refnum<vi>[])
        n256 = Build Array(w611, w609, w608, w604) -> (w610:refnum<vi>[])
        n257 = call "Enable_Disable Controls.vi"("Enable?"=TRUE, "Controls"=w606) -> ()  [unwired: 10 in]
        n258 = call "Enable_Disable Controls.vi"("Enable?"=FALSE, "Controls"=w610) -> ()  [unwired: 10 in]
      }
      frame "Set Add Unavailable" {
        n259 = Unbundle By Name(w624) -> ("Ctrl Refs.add_add"=w619:refnum<vi>, "Ctrl Refs.add_remove"=w623:refnum<vi>, "Ctrl Refs.add_Tooth"=w621:refnum<vi>, "Ctrl Refs.add_Width"=w620:refnum<vi>, "Ctrl Refs.add_Offset"=w616:refnum<vi>)
        n260 = Build Array(w619) -> (w618:refnum<vi>[])
        n261 = Build Array(w623, w621, w620, w616) -> (w622:refnum<vi>[])
        n262 = call "Enable_Disable Controls.vi"("Enable?"=TRUE, "Controls"=w618) -> ()  [unwired: 10 in]
        n263 = call "Enable_Disable Controls.vi"("Enable?"=TRUE, "Controls"=w622) -> ()  [unwired: 10 in]
      }
      frame "Refresh Add List" {
        n264 = Unbundle By Name(w631) -> ("Patterns"=w636:T3[], "Sel patterns"=w635:i32[], "Ctrl Refs.Pattern Plot"=w634:refnum<vi>, "Add List"=w628:i32, "rotations"=w627:u16)
        n265 = case shown="Default" w628 {
          selector: w628 -> [_ w643]
          tunnel: w636 -> [_ w663]
          tunnel: w635 -> [_ w662]
          tunnel: w634 -> [_ w648]
          tunnel: w633 -> [w639 w645]
          tunnel: [w639 w644] -> w632
          tunnel: [string[] ["Set Add Available"] string[] ["Set Add Unavailable", "Update Cursor Controls"]] -> w629
          tunnel: w627 -> [_ w642]
          frame -1 {
          }
          frame Default {
            # "internally teeth are zero indexed, but they are 1 indexed on GUI"
            n266 = Index Array(array=w662) -> (element=w661:i32)  [unwired: 1 in]
            n267 = Index Array(array=w663, index=w661) -> (element=w660:T3)
            n268 = Unbundle By Name(w660) -> ("Add"=w659:T6[], "Base.Length"=w655:dbl, "Base.Teeth"=w654:u16, "Base.Offset"=w653:dbl)
            n269 = Index Array(array=w659, index=w643) -> (element=w658:T6)
            n270 = Unbundle By Name(w658) -> ("Tooth"=w652:u16, "Offset"=w647:dbl, "Width"=w646:dbl)
            n271 = Divide(x=w655, y=w654) -> (x/y=w657:dbl)
            n272 = Multiply(x=w652, y=w657) -> (x*y=w656:dbl)
            n273 = Increment(x=w652) -> (x+1=w640:u16)
            n274 = Compound Arithmetic op=ADD(w656, w647, w653) -> (w651:dbl)
            n275 = local write "add_Offset"(w647) -> ()
            n276 = local write "add_Tooth"(w640) -> ()
            n277 = call "Digital Pattern Wrap Around.vi"("Rotations"=w642, "x"=w651) -> ("x"=w649:dbl)  [unwired: 9 in]
            n278 = local write "add_Width"(w646) -> ()
            n279 = property on="Property Node" class="XYGraph (strict)"(reference=w648, error in=w645, "Active Cursor"=u32 0, "Cursor.Cursor X"=w649) -> (error out=w644:errorcluster)  [unwired: 1 out]
          }
        }
        n280 = local write "Pulses Added"(w628) -> ()
        n281 = Build Array (concatenate)(w629, w637) -> (w630:string[])
      }
      frame "Refresh Remove List" {
        n282 = Unbundle By Name(w664) -> ("Rem List"=w665:i32)
        n283 = case shown="Default" w665 {
          selector: w665 -> [_ w677]
          tunnel: w669 -> [w672 w679]
          tunnel: [w672 w678] -> w668
          tunnel: [string[] ["Set Remove Available"] string[] ["Set Remove Unavailable", "Update Cursor Controls"]] -> w666
          tunnel: w664 -> [_ w676]
          frame -1 {
          }
          frame Default {
            # "internally teeth are zero indexed, but they are 1 indexed on GUI"
            n284 = Unbundle By Name(w676) -> ("Patterns"=w699:T3[], "Sel patterns"=w698:i32[], "Ctrl Refs.Pattern Plot"=w680:refnum<vi>, "rotations"=w675:u16)
            n285 = Index Array(array=w698) -> (element=w697:i32)  [unwired: 1 in]
            n286 = Index Array(array=w699, index=w697) -> (element=w696:T3)
            n287 = Unbundle By Name(w696) -> ("Base.Width"=w688:dbl, "Remove"=w695:T5[], "Base.Length"=w687:dbl, "Base.Teeth"=w686:u16, "Base.Offset"=w685:dbl)
            n288 = Index Array(array=w695, index=w677) -> (element=w694:T5)
            n289 = Unbundle By Name(w694) -> ("Tooth"=w684:u16, "Edge"=w689:bool)
            n290 = Increment(x=w684) -> (x+1=w673:u16)
            n291 = Select(t=w688, s=w689, f=sgl 0.0) -> (s? t:f=w693:dbl)
            n292 = local write "remove_Tooth"(w673) -> ()
            n293 = Divide(x=w687, y=w686) -> (x/y=w692:dbl)
            n294 = local write "Edge"(w689) -> ()
            n295 = Multiply(x=w684, y=w692) -> (x*y=w691:dbl)
            n296 = Compound Arithmetic op=ADD(w691, w693, w685) -> (w683:dbl)
            n297 = call "Digital Pattern Wrap Around.vi"("Rotations"=w675, "x"=w683) -> ("x"=w681:dbl)  [unwired: 9 in]
            n298 = property on="Property Node" class="XYGraph (strict)"(reference=w680, error in=w679, "Active Cursor"=u32 0, "Cursor.Cursor X"=w681) -> (error out=w678:errorcluster)  [unwired: 1 out]
          }
        }
        n299 = local write "Edges Removed"(w665) -> ()
        n300 = Build Array (concatenate)(w666, w670) -> (w667:string[])
      }
      frame "Hide Cursors and Edit Controls" {
        n301 = Unbundle By Name(w722) -> ("Ctrl Refs.Add List"=w721:refnum<vi>, "Ctrl Refs.Remove List"=w720:refnum<vi>, "Ctrl Refs.Pattern Name"=w719:refnum<vi>, "Ctrl Refs.remove_add"=w718:refnum<vi>, "Ctrl Refs.remove_remove"=w717:refnum<vi>, "Ctrl Refs.add_remove"=w716:refnum<vi>, "Ctrl Refs.base_Length"=w715:refnum<vi>, "Ctrl Refs.base_teeth"=w714:refnum<vi>, "Ctrl Refs.base_Toothwidth"=w713:refnum<vi>, "Ctrl Refs.base_Offset"=w712:refnum<vi>, "Ctrl Refs.add_Tooth"=w711:refnum<vi>, "Ctrl Refs.add_Width"=w710:refnum<vi>, "Ctrl Refs.add_Offset"=w709:refnum<vi>, "Ctrl Refs.remove_Tooth"=w708:refnum<vi>, "Ctrl Refs.remove_Edge"=w707:refnum<vi>, "Ctrl Refs.Chart_Position"=w706:refnum<vi>, "Ctrl Refs.Chart_Tooth"=w705:refnum<vi>, "Ctrl Refs.Chart_Offset"=w704:refnum<vi>, "Ctrl Refs.add_add"=w703:refnum<vi>, "Ctrl Refs.FPGA Resource"=w702:refnum<vi>)
        n302 = Build Array(w721, w720, w719, w718, w717, w716, w715, w714, w713, w712, w711, w710, w709, w708, w707, w706, w705, w704, w703, w702) -> (w701:refnum<vi>[])
        n303 = call "Hide_Show Controls.vi"("Hide?"=TRUE, "Controls"=w701) -> ()  [unwired: 10 in]
      }
      frame "Show Cursors and Edit Controls" {
        n304 = Unbundle By Name(w747) -> ("Ctrl Refs.Add List"=w746:refnum<vi>, "Ctrl Refs.Remove List"=w745:refnum<vi>, "Ctrl Refs.Pattern Name"=w744:refnum<vi>, "Ctrl Refs.remove_add"=w743:refnum<vi>, "Ctrl Refs.remove_remove"=w742:refnum<vi>, "Ctrl Refs.add_remove"=w741:refnum<vi>, "Ctrl Refs.base_Length"=w740:refnum<vi>, "Ctrl Refs.base_teeth"=w739:refnum<vi>, "Ctrl Refs.base_Toothwidth"=w738:refnum<vi>, "Ctrl Refs.base_Offset"=w737:refnum<vi>, "Ctrl Refs.add_Tooth"=w736:refnum<vi>, "Ctrl Refs.add_Width"=w735:refnum<vi>, "Ctrl Refs.add_Offset"=w734:refnum<vi>, "Ctrl Refs.remove_Tooth"=w733:refnum<vi>, "Ctrl Refs.remove_Edge"=w732:refnum<vi>, "Ctrl Refs.Chart_Position"=w731:refnum<vi>, "Ctrl Refs.Chart_Tooth"=w730:refnum<vi>, "Ctrl Refs.Chart_Offset"=w729:refnum<vi>, "Ctrl Refs.add_add"=w728:refnum<vi>, "Ctrl Refs.FPGA Resource"=w727:refnum<vi>)
        n305 = Build Array(w746, w745, w744, w743, w742, w741, w740, w739, w738, w737, w736, w735, w734, w733, w732, w731, w730, w729, w728, w727) -> (w726:refnum<vi>[])
        n306 = call "Hide_Show Controls.vi"("Hide?"=FALSE, "Controls"=w726) -> ()  [unwired: 10 in]
      }
      frame "Add Remove Pattern EnableDisable" {
        n307 = Unbundle By Name(w762) -> ("Patterns"=w761:T3[], "FPGA Resources"=w760:string[], "Ctrl Refs.pattern_add"=w758:refnum<vi>, "Ctrl Refs.pattern_remove"=w753:refnum<vi>)
        n308 = Array Size(array=w761) -> (size(s)=w754:i32)
        n309 = Array Size(array=w760) -> (size(s)=w759:i32)
        n310 = Greater Or Equal?(x=w754, y=w759) -> (x >= y?=w756:bool)
        n311 = Build Array(w758) -> (w757:refnum<vi>[])
        n312 = Build Array(w753) -> (w752:refnum<vi>[])
        n313 = Not(x=w756) -> (.not. x?=w755:bool)
        n314 = Equal To 0?(x=w754) -> (x = 0?=w751:bool)
        n315 = call "Enable_Disable Controls.vi"("Enable?"=w755, "Controls"=w757) -> ()  [unwired: 10 in]
        n316 = Not(x=w751) -> (.not. x?=w750:bool)
        n317 = call "Enable_Disable Controls.vi"("Enable?"=w750, "Controls"=w752) -> ()  [unwired: 10 in]
      }
      frame "<------------------ Shut Down ------------------>" {
      }
      frame "Save If Needed" {
        n318 = Unbundle By Name(w772) -> ("Need save"=w768:bool, "Node Ptr"=w770:T1, "Patterns"=w769:T3[])
        n319 = case shown="True" w768 {
          tunnel: w773 -> [w775 w779]
          tunnel: [w775 w778] -> w771
          tunnel: w770 -> [_ w777]
          tunnel: w769 -> [_ w776]
          frame False {
          }
          frame True {
            n320 = call "Save Digital Patterns.vi"("error in (no error)"=w779, "Patterns"=w776, "Item Ref in"=w777) -> ("error out"=w778:errorcluster)  [unwired: 8 in]
          }
        }
      }
      frame "SE Cleanup" {
        n321 = Unbundle By Name(w787) -> ("SE ref"=w780:refnum<vi>, "SysExp Event"=w786:refnum<event-registration>)
        n322 = Unregister For Events(event registration refnum=w786, error in=w782) -> (error out=w784:errorcluster)
        n323 = Close Reference(reference=w780, error in (no error)=w784) -> (error out=w781:errorcluster)
        n324 = invoke class="VI" method="FP.Close"(error in=w781) -> (error out=w785:errorcluster)  [unwired: 2 in, 2 out]
        n325 = call <vilib>:"NI VeriStand - Signal When Ready for Shutdown.vi"("error in (no error)"=w785) -> ("error out"=w783:errorcluster)  [unwired: 10 out]
      }
      frame "Exit" {
      }
      frame "<------------------ Macros ------------------>" {
      }
      frame "MACRO - Initialize" {
        n326 = Build Array (concatenate)(string[] ["Get SE Ref", "Get SE Event Ref", "Get Control References", "Hide Cursors and Edit Controls", "Get Persistent Data", "Get Rotations", "Select All Patterns", "Get Available FPGA Resources", "Add Remove Pattern EnableDisable", "MACRO - Refresh Patterns", "Initialize Pattern Editing", "MACRO - Refresh Lists", "Update Cursor Controls", "Release SE Cursor", "Set Init Done"], w797) -> (w796:string[])
      }
      frame "MACRO - Shut Down" {
        n327 = Build Array (concatenate)(string[] ["Save If Needed", "SE Cleanup", "Clear Busy Cursor", "Exit"], w804) -> (w803:string[])
      }
      frame "MACRO - Refresh Patterns" {
        n328 = Build Array (concatenate)(string[] ["Set Busy Cursor", "Populate Patterns List", "Plot Pattern(s)", "Clear Busy Cursor"], w809) -> (w808:string[])
      }
      frame "MACRO - Refresh Lists" {
        n329 = Build Array (concatenate)(string[] ["Refresh Remove List", "Refresh Add List"], w814) -> (w813:string[])
      }
      frame "<------------------ Initialization ------------------>" {
      }
      frame "Get Control References" {
        n330 = control-ref of="Pattern Plot"() -> (w843:refnum<vi>)
        n331 = control-ref of="remove_add"() -> (w837:refnum<vi>)
        n332 = control-ref of="remove_remove"() -> (w836:refnum<vi>)
        n333 = control-ref of="add_remove"() -> (w835:refnum<vi>)
        n334 = control-ref of="Edge"() -> (w827:refnum<vi>)
        n335 = control-ref of="add_add"() -> (w823:refnum<vi>)
        n336 = control-ref of="pattern_remove"() -> (w822:refnum<vi>)
        n337 = control-ref of="pattern_add"() -> (w821:refnum<vi>)
        n338 = control-ref of="Header"() -> (w844:refnum<vi>)
        n339 = control-ref of="Patterns"() -> (w841:refnum<vi>)
        n340 = control-ref of="Pulses Added"() -> (w840:refnum<vi>)
        n341 = control-ref of="Edges Removed"() -> (w839:refnum<vi>)
        n342 = control-ref of="base_Length"() -> (w834:refnum<vi>)
        n343 = control-ref of="base_teeth"() -> (w819:refnum<vi>)
        n344 = control-ref of="base_Toothwidth"() -> (w833:refnum<vi>)
        n345 = control-ref of="base_Offset"() -> (w832:refnum<vi>)
        n346 = control-ref of="add_Tooth"() -> (w831:refnum<vi>)
        n347 = control-ref of="add_Width"() -> (w830:refnum<vi>)
        n348 = control-ref of="add_Offset"() -> (w829:refnum<vi>)
        n349 = control-ref of="remove_Tooth"() -> (w828:refnum<vi>)
        n350 = control-ref of="Chart_Position"() -> (w826:refnum<vi>)
        n351 = control-ref of="Chart_Tooth"() -> (w825:refnum<vi>)
        n352 = control-ref of="Chart_Offset"() -> (w824:refnum<vi>)
        n353 = control-ref of="Pattern Name"() -> (w838:refnum<vi>)
        n354 = control-ref of="Zoom"() -> (w842:refnum<vi>)
        n355 = control-ref of="FPGA Resource"() -> (w820:refnum<vi>)
        n356 = Bundle By Name(cluster=w848, "Ctrl Refs.Header"=w844, "Ctrl Refs.Pattern Plot"=w843, "Ctrl Refs.Zoom"=w842, "Ctrl Refs.Select Pattern"=w841, "Ctrl Refs.Add List"=w840, "Ctrl Refs.Remove List"=w839, "Ctrl Refs.Pattern Name"=w838, "Ctrl Refs.remove_add"=w837, "Ctrl Refs.remove_remove"=w836, "Ctrl Refs.add_remove"=w835, "Ctrl Refs.base_Length"=w834, "Ctrl Refs.base_teeth"=w819, "Ctrl Refs.base_Toothwidth"=w833, "Ctrl Refs.base_Offset"=w832, "Ctrl Refs.add_Tooth"=w831, "Ctrl Refs.add_Width"=w830, "Ctrl Refs.add_Offset"=w829, "Ctrl Refs.remove_Tooth"=w828, "Ctrl Refs.remove_Edge"=w827, "Ctrl Refs.Chart_Position"=w826, "Ctrl Refs.Chart_Tooth"=w825, "Ctrl Refs.Chart_Offset"=w824, "Ctrl Refs.add_add"=w823, "Ctrl Refs.pattern_remove"=w822, "Ctrl Refs.pattern_add"=w821, "Ctrl Refs.FPGA Resource"=w820) -> (w847:T2)
      }
      frame "Release SE Cursor" {
        n357 = call <vilib>:"NI VeriStand - Unset Busy Cursor.vi"("error in (no error)"=w850) -> ("error out"=w849:errorcluster)  [unwired: 10 out]
      }
      frame "Get SE Event Ref" {
        n358 = call <vilib>:"NI VeriStand - Get Event Refnum.vi"("error in (no error)"=w857) -> ("error out"=w858:errorcluster, "Event Ref"=w859:refnum<user-event>)  [unwired: 9 out]
        n359 = register-events(error in=w858, w859) -> (reference out=w854:refnum<event-registration>, error out=w856:errorcluster)  [unwired: 1 in]
        n360 = Bundle By Name(cluster=w855, "SysExp Event"=w854) -> (w853:T2)
      }
      frame "Get SE Ref" {
        n361 = Open VI Reference(vi path="System Explorer.lvlib:System Explorer.vi" ("Separator (,)"), error in (no error)=w864) -> (vi reference=w861:refnum<vi>, error out=w863:errorcluster)  [unwired: 4 in]
        n362 = Bundle By Name(cluster=w866, "SE ref"=w861) -> (w862:T2)
      }
      frame "Set Init Done" {
        n363 = Bundle By Name(cluster=w870, "Init done"=TRUE) -> (w869:T2)
      }
      frame "Get Persistent Data" {
        n364 = Unbundle By Name(w877) -> ("Node Ptr"=w876:T1)
        n365 = call "Get Digital Patterns.vi"("error in (no error)"=w878, "Item Ref in"=w876) -> ("error out"=w874:errorcluster, "Patterns"=w873:T3[])  [unwired: 7 in, 1 out]
        n366 = Bundle By Name(cluster=w877, "Patterns"=w873) -> (w875:T2)
      }
      frame "Get Rotations" {
        n367 = Unbundle By Name(w893) -> ("Ctrl Refs.Zoom"=w886:refnum<vi>, "Node Ptr"=w881:T1)
        n368 = call "Get APU Characteristics.vi"("error in (no error)"=w894, "Item Ref in"=w881) -> ("error out"=w882:errorcluster, "rotations"=w880:u16)  [unwired: 3 in, 5 out]
        n369 = Bundle By Name(cluster=w893, "rotations"=w880) -> (w892:T2)
        n370 = Multiply(x=w880, y=180.0 ("t")) -> (x*y=w890:dbl)
        n371 = Negate(x=w890) -> (-x=w891:dbl)
        n372 = property on="Property Node" class="Slide (strict)"(reference=w886, error in=w882, "Scale.Maximum"=w890, "Maximum"=w890, "Minimum"=w891, "Scale.Minimum"=w891) -> (reference out=w885:refnum<vi>, error out=w884:errorcluster, "Value"=w888:cluster{dbl, dbl})
        n373 = Bundle(cluster=w888, w890, w891) -> (w889:cluster{dbl, dbl})
        n374 = property on="Property Node" class="Slide (strict)"(reference=w885, error in=w884, "Val(Sgnl)"=w889) -> (error out=w883:errorcluster)  [unwired: 1 out]
      }
      frame "Get Available FPGA Resources" {
        n375 = Unbundle By Name(w904) -> ("Ctrl Refs.FPGA Resource"=w899:refnum<vi>, "Node Ptr"=w903:T1)
        n376 = global read "Properties.vi" "Main.Digital PatGens"() -> (w902:string)
        n377 = global read "Constants and GUIDs.vi" "Constant.Pick FPGA resource"() -> (w898:string)
        n378 = call "Get Available IP List.vi"("ip list property name"=w902, "error in (no error)"=w906, "Item Ref in"=w903) -> ("error out"=w905:errorcluster, "ips available"=w897:string[])  [unwired: 6 in, 1 out]
        n379 = Build Array (concatenate)(w898, w897) -> (w896:string[])
        n380 = Bundle By Name(cluster=w904, "FPGA Resources"=w897) -> (w901:T2)
        n381 = property class="Ring (strict)"(reference=w899, error in=w905, "Strings []"=w896) -> (error out=w900:errorcluster)  [unwired: 1 out]
      }
      frame "Select All Patterns" {
        n382 = Unbundle By Name(w912) -> ("Patterns"=w911:T3[])
        n383 = Array Size(array=w911) -> (size(s)=w909:i32)
        n384 = for {
          N: w909 -> [_]
          tunnel: [w915] -> w908 mode=indexing
          i -> [w915]
        }
        n385 = Bundle By Name(cluster=w912, "Sel patterns"=w908) -> (w910:T2)
      }
      frame "Initialize Pattern Editing" {
        n386 = Unbundle By Name(w917) -> ("Sel patterns"=w921:i32[])
        n387 = Array Size(array=w921) -> (size(s)=w918:i32)
        n388 = case shown="1" w918 {
          tunnel: w920 -> [w924 w927]
          tunnel: [w923 w926] -> w919
          frame 1 {
            n389 = Build Array (concatenate)(string[] ["Update Pattern Controls", "Show Cursors and Edit Controls"], w924) -> (w923:string[])
          }
          frame Default {
            n390 = Build Array (concatenate)(string[] ["Hide Cursors and Edit Controls"], w927) -> (w926:string[])
          }
        }
      }
    }
    n391 = case shown="Error" w10 {
      tunnel: w15 -> [w19 w20]
      tunnel: [w19 w21] -> w13
      frame No Error {
      }
      frame Error {
        n392 = Build Array (concatenate)("Error", w20) -> (w21:string[])
      }
    }
  }
  "error out" <- w5
